vi "Classes Destruction.vi"(7 "class labels":T1, 8 "error in":errorcluster, 11 "classes in":T2) -> (0 "error out":errorcluster, 3 "classes out":T2)   [LabVIEW 2011]
uses:
  Controls/Class Objects.ctl
  Modules/File/Configuration/Configuration.lvclass
  Modules/Hardware/Power Supply/Power Supply.lvclass
  Modules/Hardware/Mass Flow Controller/Mass Flow Controller.lvclass
  Modules/Hardware/Detector/Detector.lvclass
  Modules/File/TDMS/TDMS.lvclass
  Controls/Class Labels.ctl
  Functional Globals/Device Parameters.ctl
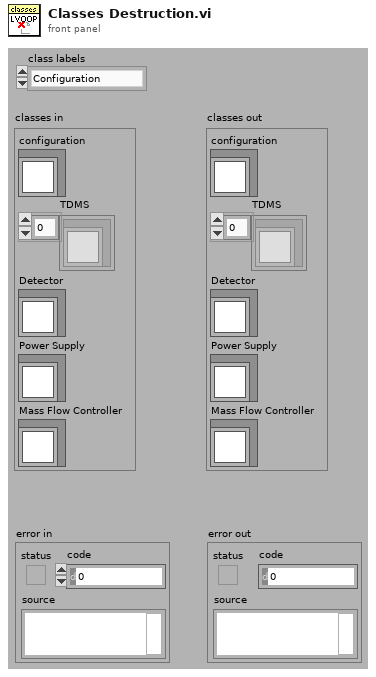
[diagram p1: front panel]
types:
  T1 = typedef "Class Labels.ctl" = enum16{"Configuration", "TDMS", "Detector", "Power Supply", "MFC", "NMR", "Valve Controller"}
  T2 = typedef "Class Objects.ctl" = cluster{"configuration":refnum<class "Configuration.lvclass">, "TDMS":refnum<class "TDMS.lvclass">[], "Power Supply":refnum<class "Power Supply.lvclass">, "Mass Flow Controller":refnum<class "Mass Flow Controller.lvclass">, "Detector":refnum<class "Detector.lvclass">}
  T3 = typedef "Device Parameters.ctl" = enum16{"Initialize", "Set Device Connections", "Set Device Settings", "Get Device Connections", "Get Device Settings"}
  T4 = typedef "Device Connections.ctl" = cluster{"Device Name":cluster{"VISA resource name":refnum<visa-resource-name>}}
  T5 = typedef "Device Settings.ctl" = cluster{"Device Name":cluster{"Setpoint":dbl}}
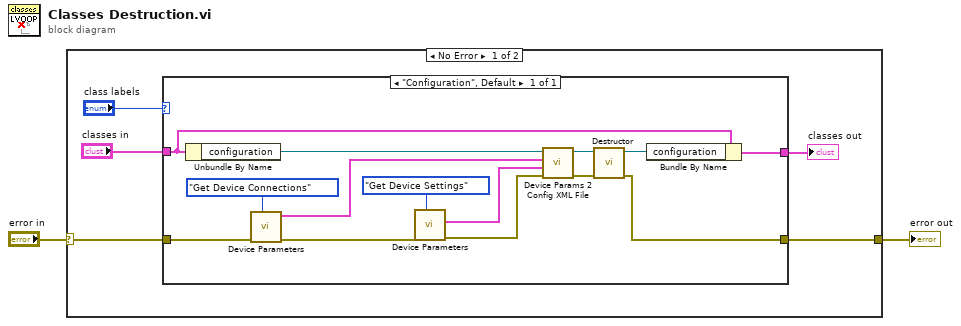
[diagram p0: block diagram]
diagram:
  n1 = case shown="No Error" "error in" {
    selector: "error in" -> [w5 w22]
    tunnel: [w3 w22] -> w1
    frame No Error {
      n2 = case shown="\"Configuration\", Default" "class labels" {
        tunnel: "classes in" -> [w21]
        tunnel: w5 -> [w14]
        tunnel: [w19] -> w3
        tunnel: [w18] -> w4
        frame "Configuration", Default {
          n3 = Unbundle By Name(w21) -> ("configuration"=w16:refnum<class "Configuration.lvclass">)
          n4 = call "Device Parameters.vi"("command"=Device_Parameters."Get Device Connections", "error in"=w14) -> ("error out"=w11:errorcluster, "Device Connections OUT"=w10:T4)  [unwired: 7 in, 1 out]
          n5 = call "Device Parameters.vi"("command"=Device_Parameters."Get Device Settings", "error in"=w11) -> ("error out"=w8:errorcluster, "Device Settings OUT"=w9:T5)  [unwired: 7 in, 1 out]
          n6 = call "Device Params 2 Config XML File.vi"("error IN"=w8, "Device Settings"=w9, "Device Connections"=w10, "Configuration in"=w16) -> ("error OUT"=w17:errorcluster, "Configuration out"=w15:refnum<class "Configuration.lvclass">)  [unwired: 6 in]
          n7 = call-dynamic "Destructor.vi"("error in (no error)"=w17, "Configuration in"=w15) -> ("error out"=w19:errorcluster, "Configuration out"=w20:refnum<class "Configuration.lvclass">)  [unwired: 8 in]
          n8 = Bundle By Name(cluster=w21, "configuration"=w20) -> (w18:T2)
        }
      }
      "classes out" <- w4
    }
    frame Error {
    }
  }
  "error out" <- w1
